vi "Layer Scan V5.vi"() -> ()   [LabVIEW 2024]
uses:
  <vilib>/DAQmx/write.llb/DAQmx Write (Analog 1D DBL NChan 1Samp).vi
  <vilib>/DAQmx/create/channels.llb/DAQmx Create Channel (AO-Voltage-Basic).vi
  <vilib>/DAQmx/miscellaneous.llb/DAQmx Fill In Error Info.vi
  <instrlib>/niScope/Utility/niScope Get Channel Name From String.vi
  <instrlib>/niScope/Configure/Trigger/niScope Configure Trigger Immediate.vi
  <instrlib>/niScope/Configure/Trigger/niScope Configure Trigger Edge.vi
  <instrlib>/niScope/Configure/Trigger/niScope Configure Trigger Digital.vi
  <instrlib>/niScope/Configure/Trigger/niScope Configure Trigger Window.vi
  <instrlib>/niScope/Configure/Trigger/niScope Configure Trigger Hysteresis.vi
  <instrlib>/niScope/Acquire/Fetch/niScope Fetch Cluster.vi
  <vilib>/express/express analysis/Spectral/Block/exnSpectralBlock spectral measurements peak poly.vi
  <vilib>/express/express analysis/Spectral/Block/exnSpectralBlock spectral measurements peak WFM.vi
  <vilib>/express/express analysis/Spectral/XNode/ExpressSpectralMeasurementsBlockNode.xnode
panel:
  out "FFT Graph":cluster{"f0":dbl, "df":dbl, "magnitude":dbl[]}(graph)
  in  "Resource Name":refnum<k15>="Dev1" caption="Resource Name(s)"
  in  "Simulate?":bool
  in  "Channel Name":string="0" caption="Channel(s)"
  in  "Enforce Realtime":bool=TRUE
  in  "Vertical Range":dbl=5.0 caption="Vertical Range (V)" format="%.2f"
  in  "Min Sample Rate":dbl=10000000.0 caption="Min. Sample Rate" step=1000000.0 format="%#.2p"
  in  "Min Record Length":i32=1000 caption="Min. Record Length"
  out "Waveform(s)":T1(graph)
  out "Actual Record Length":i32=1000
  out "Actual Sample Rate":dbl=10000000.0 format="%#.2p"
  in  "Timeout (s)":dbl=5.0 caption="Timeout(s)" format="%.2f"
  in  "Vertical Offset":dbl caption="Vertical Offset (V)" format="%.2p"
  in  "Probe Attenuation":dbl=1.0 format="%.1f"
  in  "Input Impedance":u32(ring) items=["1 mega ohm"=0, "50 ohms"=2]
  in  "Maximum Input Frequency":dbl caption="Max. Input Frequency (Hz)" format="%.2f"
  in  "Trigger Delay":dbl caption="Trigger Delay (s)" format="%#.4p"
  in  "Reference Position":dbl=50.0 caption="Ref Position" format="%.1f"
  in  "Stop":bool
  in  "Vertical Coupling":i32(ring)=1 items=["AC", "DC", "Ground"]
  in  "Trigger Modifier":i32(ring)=2 items=["None"=1, "Auto Trigger"=2]
  out "Auto Triggered":bool
  in  "Trigger Type":T2(tab)
  in  "Trigger Source":string(combo)="0"
  in  "Trigger Level":dbl format="%.2f"
  in  "Trigger Slope":i32(ring) items=["Positive", "Negative"]
  in  "Coupling":u16(ring)=1 caption="Trigger Coupling" items=["AC"=0, "DC"=1, "HF Reject"=3, "LF Reject"=4, "AC Plus HF Reject"=1001]
  in  "Trigger Slope 2":i32(ring) caption="Trigger Slope" items=["Positive", "Negative"]
  in  "Trigger Source 2":string(combo)="VAL_PFI_1" caption="Trigger Source"
  in  "Coupling 2":u16(ring)=1 caption="Trigger Coupling" items=["AC"=0, "DC"=1, "HF Reject"=3, "LF Reject"=4, "AC Plus HF Reject"=1001]
  in  "High Level":dbl=0.1 caption="Window High Level" format="%.2f"
  in  "Low Level":dbl=-0.1 caption="Window Low Level" format="%.2f"
  in  "Window Mode":i32(ring) items=["Entering", "Leaving"]
  in  "Trigger Source 3":string(combo)="0" caption="Trigger Source"
  in  "Hysteresis":dbl=0.05 format="%.2f"
  in  "Trigger Source 4":string(combo)="0" caption="Trigger Source"
  in  "Trigger Level 2":dbl caption="Trigger Level" format="%.2f"
  in  "Coupling 3":u16(ring)=1 caption="Trigger Coupling" items=["AC"=0, "DC"=1, "HF Reject"=3, "LF Reject"=4, "AC Plus HF Reject"=1001]
  in  "Trigger Slope 3":i32(ring) caption="Trigger Slope" items=["Positive", "Negative"]
  out "decimated array 2":dbl[](array[numeric])
  out "decimated array":dbl[](array[numeric])
  out "Y coord filename":i32
  out "x coord file name":i32
  out "Filename Out":path
  in  "Data File Name":path
  in  "Data folder Path":path
  in  "X offset":dbl
  in  "Y offset":dbl
  in  "distance":dbl
  in  "Y Count":dbl
  in  "X Count":dbl
  # "Note: When configured for Immediate reference trigger, this example does not configure any additional trigger settings - the acquisition is triggered as soon as possible after being initiated by driver software."
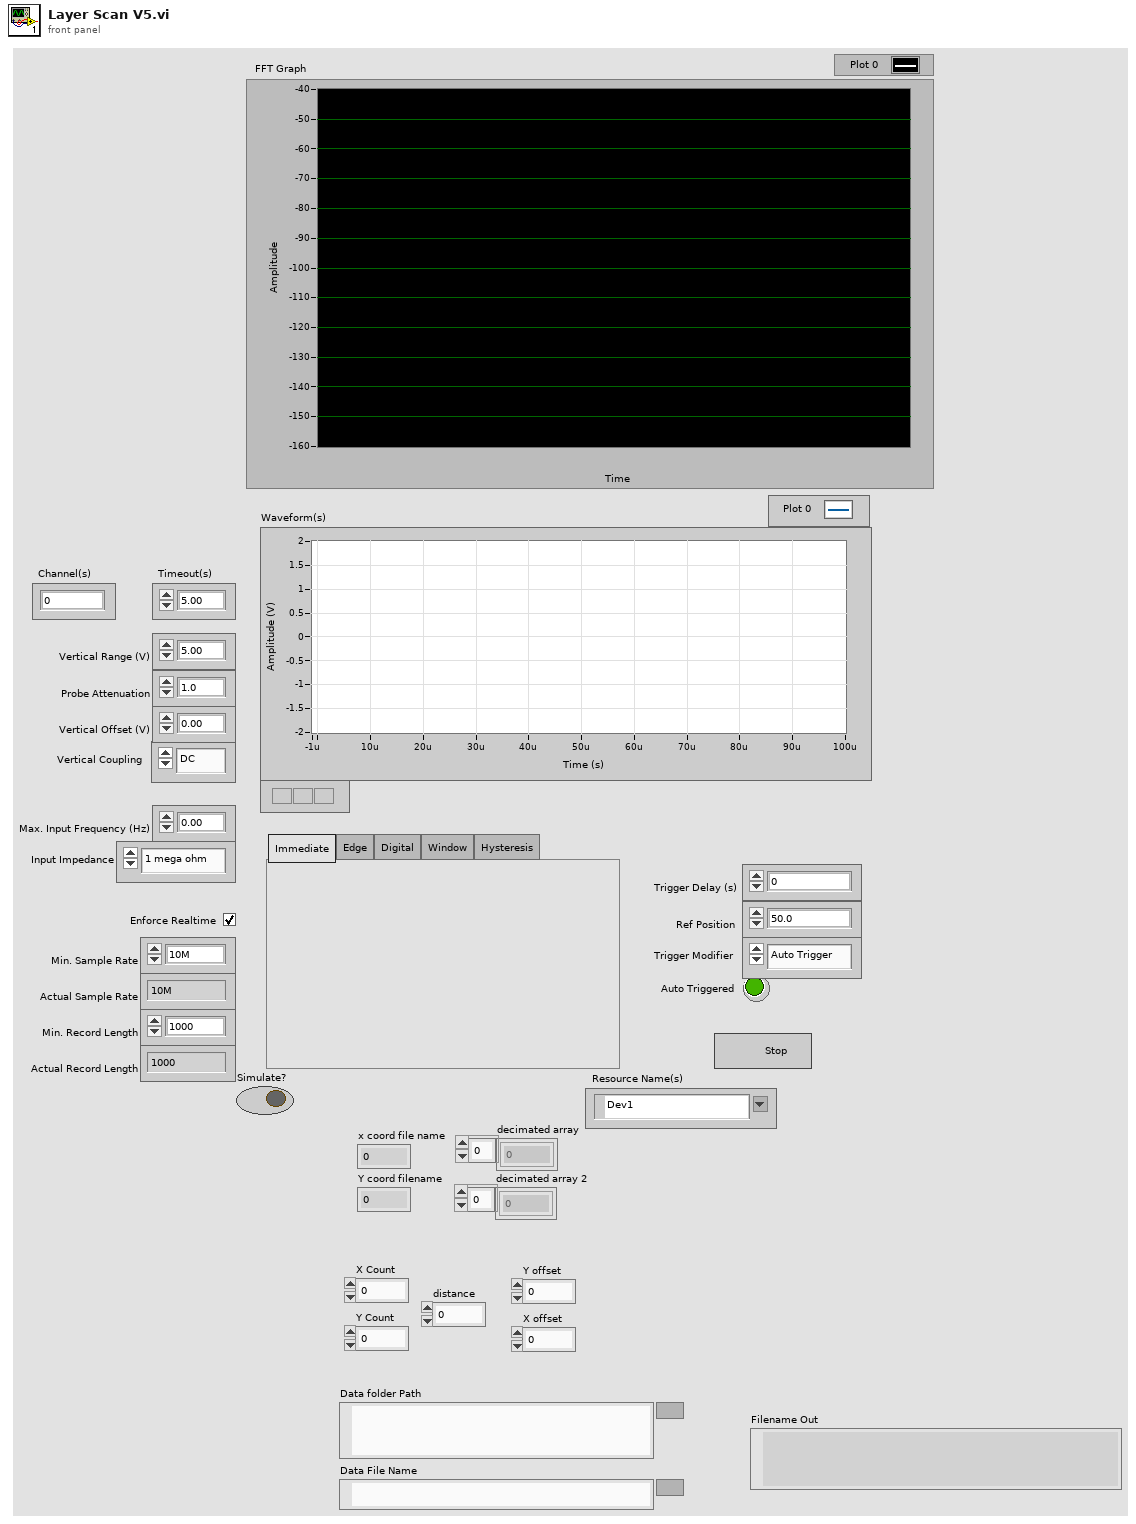
[diagram p1: front panel]
types:
  T1 = cluster{"relativeInitialX":dbl, "xIncrement":dbl, "wfm":dbl[]}
  T2 = enum32{"Immediate", "Edge", "Digital", "Window", "Hysteresis"}
  T3 = cluster{"averaging mode":u16, "weighting mode":u16, "number of averages":u32}
  T4 = cluster{"dB On (F)":bool, "unwrap phase (F)":bool, "convert to degree (F)":bool}
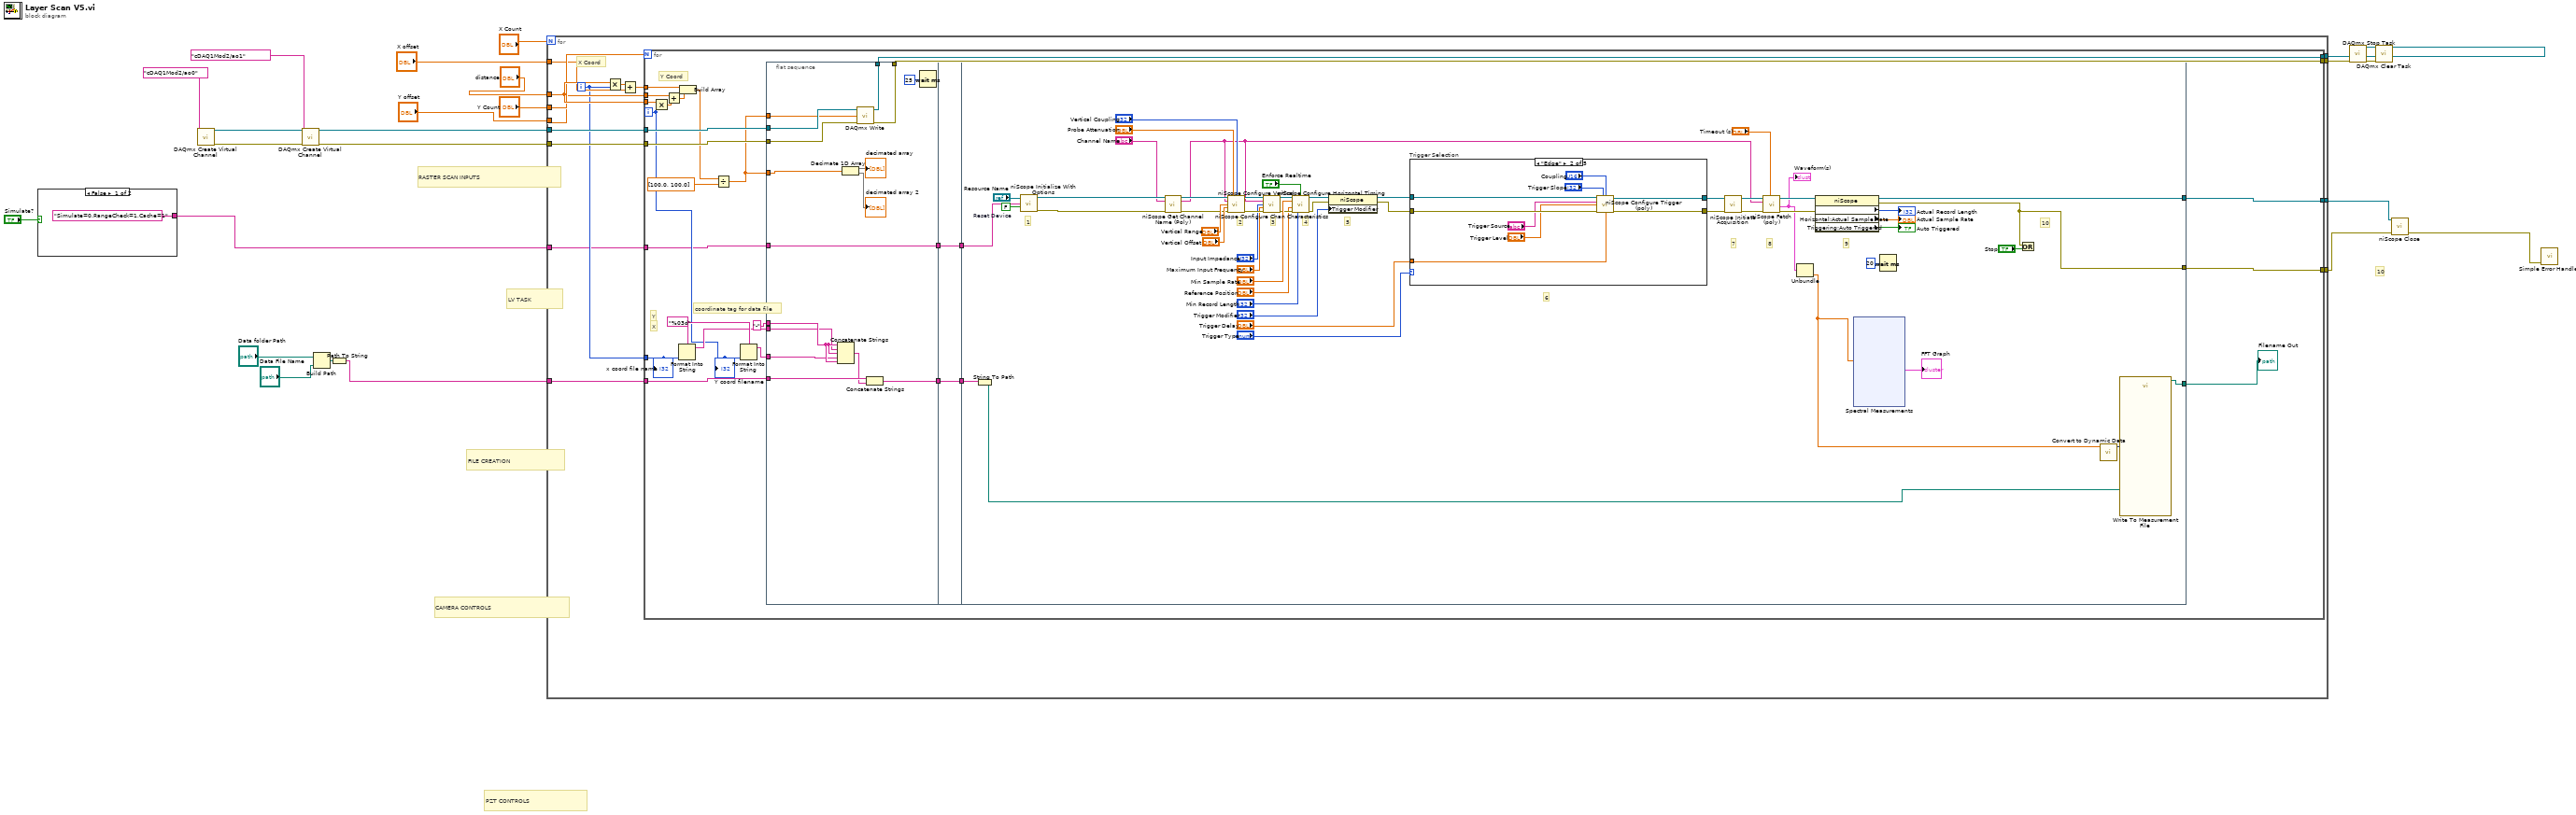
[diagram p0: block diagram]
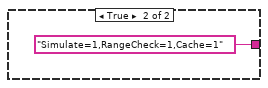
[diagram p2: hidden frame]
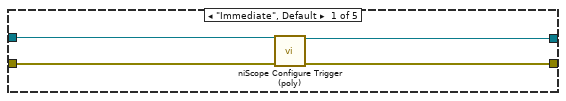
[diagram p3: hidden frame]
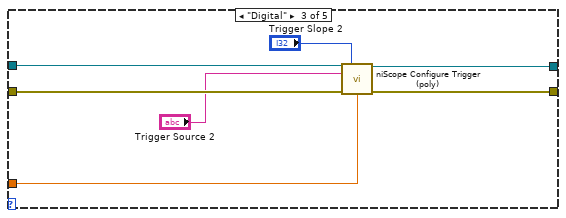
[diagram p4: hidden frame]
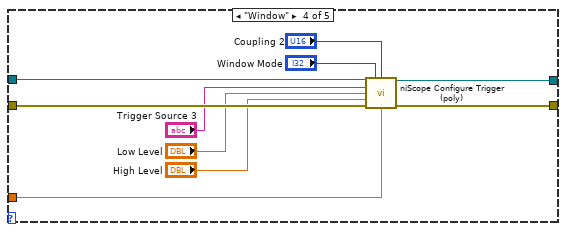
[diagram p5: hidden frame]
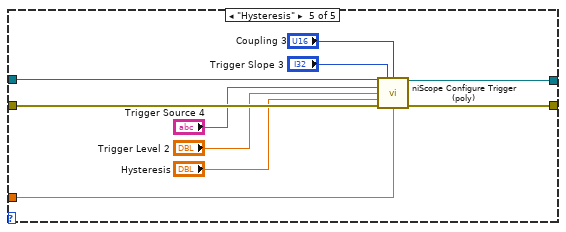
[diagram p6: hidden frame]
diagram:
  # "10"
  # "FILE CREATION"
  # "PZT CONTROLS"
  # "CAMERA CONTROLS"
  # "LV TASK"
  # "RASTER SCAN INPUTS"
  n1 = case shown="False" "Simulate?" {
    tunnel: ["Simulate=0,RangeCheck=1,Cache=1" ("option string") "Simulate=1,RangeCheck=1,Cache=1" ("option string")] -> w1
    frame False {
    }
    frame True {
    }
  }
  n2 = call-poly <vilib>:"DAQmx Create Virtual Channel.vi"("physical channels"=tag "cDAQ1Mod2/ao0") -> ("task out"=w17:refnum<k21>, "error out"=w16:errorcluster)  [unwired: 13 in]
  n3 = call-poly <vilib>:"DAQmx Create Virtual Channel.vi"("task in"=w17, "physical channels"=tag "cDAQ1Mod2/ao1", "error in"=w16) -> ("task out"=w15:refnum<k21>, "error out"=w14:errorcluster)  [unwired: 11 in]
  n4 = Build Path(base path="Data folder Path", name or relative path="Data File Name") -> (appended path=w7:path)
  n5 = Path To String(path=w7) -> (string=w6:string)
  n6 = for {
    N: "X Count" -> [_]
    tunnel: "distance" -> [w41]
    tunnel: "Y Count" -> [w40]
    tunnel: "Y offset" -> [w39]
    tunnel: "X offset" -> [w37]
    tunnel: w15 -> [w35]
    tunnel: w14 -> [w34]
    tunnel: [w33] -> w13
    tunnel: [w32] -> w12
    tunnel: [w31] -> w4
    tunnel: w6 -> [w30]
    tunnel: w1 -> [w28]
    tunnel: [w27] -> w5
    i -> [w29]
    # "X Coord"
    n7 = Multiply(x=w41, y=w29) -> (x*y=w38:dbl)
    n8 = Add(x=w38, y=w37) -> (x+y=w36:dbl)
    n9 = for {
      N: w40 -> [_]
      tunnel: w41 -> [w68]
      tunnel: w39 -> [w66]
      tunnel: w36 -> [w65]
      tunnel: w35 -> [w63]
      tunnel: w34 -> [w62]
      tunnel: [w60] -> w33
      tunnel: [w59] -> w32
      tunnel: [w47] -> w31
      tunnel: w30 -> [w54]
      tunnel: w29 -> [w50]
      tunnel: w28 -> [w43]
      tunnel: [w42] -> w27
      i -> [w49]
      w58 = "%03d" ("format string")
      # "coordinate tag for data file"
      # "X"
      # "Y"
      # "Y Coord"
      n10 = Multiply(x=w68, y=w49) -> (x*y=w67:dbl)
      n11 = Add(x=w66, y=w67) -> (x+y=w64:dbl)
      n12 = Format Into String(format string=w58, w50) -> (resulting string=w56:string)  [unwired: 2 in, 1 out]
      n13 = Build Array(w65, w64) -> (w61:dbl[])
      n14 = Divide(x=w61, y=dbl[] [100.0, 100.0]) -> (x/y=w48:dbl[])
      n15 = Format Into String(format string=w58, w49) -> (resulting string=w55:string)  [unwired: 2 in, 1 out]
      n16 = flat-sequence {
        tunnel: w63 -> [w83]
        tunnel: w62 -> [w82]
        tunnel: [w81] -> w60
        tunnel: [w80] -> w59
        tunnel: "-" ("string") -> [w79]
        tunnel: w56 -> [w78]
        tunnel: w55 -> [w77]
        tunnel: w54 -> [w76]
        tunnel: [w74] -> w53
        tunnel: w48 -> [w73]
        tunnel: w48 -> [w72]
        tunnel: [w69] -> w45
        tunnel: w43 -> [w69]
        tunnel: w53 -> [w86]
        tunnel: [w86] -> w52
        tunnel: w45 -> [w85]
        tunnel: [w85] -> w44
        tunnel: w52 -> [w129]
        tunnel: [w136] -> w47
        tunnel: [w137] -> w46
        tunnel: w44 -> [w131]
        tunnel: [w135] -> w42
        frame #0 {
          n17 = Concatenate Strings(w79, w78, w79, w77, w79) -> (w75:string)
          n18 = Decimate 1D Array(w72) -> (→"decimated array":dbl[], →"decimated array 2":dbl[])
          n19 = call-poly <vilib>:"DAQmx Write.vi"("task/channels in"=w83, "data"=w73, "error in"=w82) -> ("task out"=w81:refnum<k21>, "error out"=w80:errorcluster)  [unwired: 10 in, 1 out]
          n20 = Concatenate Strings(w76, w75) -> (w74:string)
          n21 = Wait (ms)(milliseconds to wait=u32 25) -> ()  [unwired: 1 out]
        }
        frame #1 {
        }
        frame #2 {
          w134 = FALSE  # Reset Device
          # "5"
          # "2"
          # "3"
          # "4"
          # "6"
          # "7"
          # "8"
          # "9"
          # "10"
          # "1"
          n22 = String To Path(string=w129) -> (path=w128:path)
          n23 = call <instrlib>:"niScope Initialize With Options.vi"("resource name"="Resource Name", "option string"=w131, "reset device"=w134) -> ("instrument handle"=w130:refnum<k15>, "error out"=w132:errorcluster)  [unwired: 11 in]
          n24 = call-poly <instrlib>:"niScope Get Channel Name (Poly).vi"("instrument handle"=w130, "index"="Channel Name", "error in"=w132) -> ("instrument handle out"=w94:refnum<k15>, "channel name"=w91:string, "error out"=w93:errorcluster)  [unwired: 10 in]
          n25 = call <instrlib>:"niScope Configure Vertical.vi"("instrument handle"=w94, "probe attenuation"="Probe Attenuation", "vertical coupling"="Vertical Coupling", "channels"=w91, "vertical range"="Vertical Range", "vertical offset"="Vertical Offset", "error in"=w93) -> ("instrument handle out"=w124:refnum<k15>, "error out"=w123:errorcluster)  [unwired: 7 in]
          n26 = call <instrlib>:"niScope Configure Chan Characteristics.vi"("instrument handle"=w124, "channels"=w91, "input impedance"="Input Impedance", "maximum input frequency"="Maximum Input Frequency", "error in"=w123) -> ("instrument handle out"=w121:refnum<k15>, "error out"=w122:errorcluster)  [unwired: 9 in]
          n27 = call <instrlib>:"niScope Configure Horizontal Timing.vi"("instrument handle"=w121, "enforce realtime"="Enforce Realtime", "min sample rate"="Min Sample Rate", "reference position"="Reference Position", "error in"=w122, "min record length"="Min Record Length") -> ("instrument handle out"=w106:refnum<k15>, "error out"=w105:errorcluster)  [unwired: 8 in]
          n28 = property on="Property Node" class="niScope"(reference=w106, error in=w105, "Trigger Modifier"="Trigger Modifier") -> (reference out=w103:refnum<k15>, error out=w104:errorcluster)
          n29 = case "Trigger Selection" shown="\"Edge\"" "Trigger Type" {
            tunnel: w104 -> [w151 w160 w167 w177 w187]
            tunnel: [w148 w156 w163 w173 w183] -> w109
            tunnel: w103 -> [w150 w159 w166 w176 w186]
            tunnel: [w149 w157 w164 w174 w185] -> w112
            tunnel: "Trigger Delay" -> [_ w158 w165 w175 w184]
            frame "Immediate", Default {
              n30 = call-poly <instrlib>:"niScope Configure Trigger (poly).vi"("instrument handle"=w150, "error in"=w151) -> ("instrument handle out"=w149:refnum<k15>, "error out"=w148:errorcluster)  [unwired: 12 in]
            }
            frame "Edge" {
              n31 = call-poly <instrlib>:"niScope Configure Trigger (poly).vi"("instrument handle"=w159, "trigger slope"="Trigger Slope", "trigger coupling"="Coupling", "trigger source"="Trigger Source", "trigger level"="Trigger Level", "error in"=w160, "trigger delay"=w158) -> ("instrument handle out"=w157:refnum<k15>, "error out"=w156:errorcluster)  [unwired: 7 in]
            }
            frame "Digital" {
              n32 = call-poly <instrlib>:"niScope Configure Trigger (poly).vi"("instrument handle"=w166, "trigger slope"="Trigger Slope 2", "trigger source"="Trigger Source 2", "error in"=w167, "trigger delay"=w165) -> ("instrument handle out"=w164:refnum<k15>, "error out"=w163:errorcluster)  [unwired: 9 in]
            }
            frame "Window" {
              n33 = call-poly <instrlib>:"niScope Configure Trigger (poly).vi"("instrument handle"=w176, "trigger window mode"="Window Mode", "trigger coupling"="Coupling 2", "trigger source"="Trigger Source 3", "low level"="Low Level", "high level"="High Level", "error in"=w177, "trigger delay"=w175) -> ("instrument handle out"=w174:refnum<k15>, "error out"=w173:errorcluster)  [unwired: 6 in]
            }
            frame "Hysteresis" {
              n34 = call-poly <instrlib>:"niScope Configure Trigger (poly).vi"("instrument handle"=w186, "trigger slope"="Trigger Slope 3", "trigger coupling"="Coupling 3", "trigger source"="Trigger Source 4", "trigger level"="Trigger Level 2", "hysteresis"="Hysteresis", "error in"=w187, "trigger delay"=w184) -> ("instrument handle out"=w185:refnum<k15>, "error out"=w183:errorcluster)  [unwired: 6 in]
            }
          }
          n35 = call <instrlib>:"niScope Initiate Acquisition.vi"("instrument handle"=w112, "error in"=w109) -> ("instrument handle out"=w111:refnum<k15>, "error out"=w110:errorcluster)  [unwired: 12 in]
          n36 = call-poly <instrlib>:"niScope Fetch (poly).vi"("timeout"="Timeout (s)", "error in"=w110, "channels"=w91, "instrument handle"=w111) -> ("error out"=w100:errorcluster, "waveform"=w90:T1, "instrument handle out"=w101:refnum<k15>)  [unwired: 4 in, 1 out]
          "Waveform(s)" <- w90
          n37 = Unbundle(w90) -> ("wfm"=w88:dbl[])  [unwired: 2 out]
          n38 = property class="niScope"(reference=w101, error in=w100) -> (reference out=w135:refnum<k15>, error out=w136:errorcluster, "Horizontal:Actual Record Length"=→"Actual Record Length":i32, "Horizontal:Actual Sample Rate"=→"Actual Sample Rate":dbl, "Triggering:Auto Triggered"=→"Auto Triggered":bool)
          n39 = xnode "Spectral Measurements"("Signals"=w88) -> ("FFT - (Peak)"=→"FFT Graph":cluster{"f0":dbl, "df":dbl, "magnitude":dbl[]})  [unwired: 1 in, 2 out]
          n40 = Wait (ms)(milliseconds to wait=u32 20) -> ()  [unwired: 1 out]
          n41 = Or(x=w136, y="Stop") -> ()  [unwired: 1 out]
          n42 = call "Convert to Dynamic Data"("Array"=w88) -> ("Dynamic Data Type"=w89:dynamicdata)  [unwired: 3 in]
          n43 = call "Write To Measurement File"("Signals"=w89, "Filename"=w128) -> ("Filename Out"=w137:path)  [unwired: 15 in, 2 out]
        }
      }
      "Filename Out" <- w46
      "x coord file name" <- w50
      "Y coord filename" <- w49
    }
  }
  n44 = call <vilib>:"DAQmx Stop Task.vi"("task/channels in"=w13, "error in"=w12) -> ("task out"=w11:refnum<k21>, "error out"=w10:errorcluster)  [unwired: 12 in]
  n45 = call <vilib>:"DAQmx Clear Task.vi"("task in"=w11, "error in"=w10) -> ()  [unwired: 13 in, 1 out]
  n46 = call <instrlib>:"niScope Close.vi"("instrument handle"=w5, "error in"=w4) -> ("error out"=w3:errorcluster)  [unwired: 13 in]
  n47 = call <vilib>:"Simple Error Handler.vi"("error in (no error)"=w3) -> ()  [unwired: 4 in, 5 out]
